vi "Stop All Channels streaming.vi"(1 "Template Refs":refnum<vi>[](array[refnum]), 2 "Handle":i32, 3 "LMMeasurementLib.ICoLMMeasurement":refnum<k7>) -> (0 "error out":errorcluster)   [LabVIEW 2017, in "Powermeter_library.lvlib"]
uses:
  Powermeter_library.lvlib
  Channel States.ctl
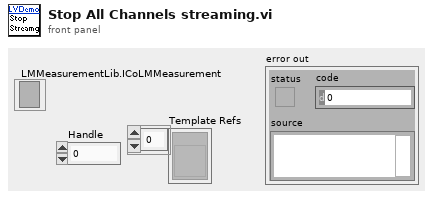
[diagram p1: front panel]
types:
  T1 = typedef "Powermeter_library.lvlib/Channel States.ctl" = enum16{"Init", "Poll", "Set Handle", "Measure"}
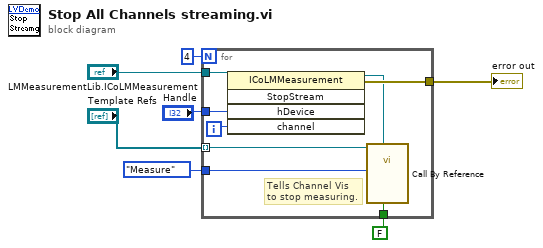
[diagram p0: block diagram]
diagram:
  n1 = for {
    N: 4 -> [_]
    tunnel: "LMMeasurementLib.ICoLMMeasurement" -> [w15]
    tunnel: "Handle" -> [w14]
    tunnel: [w13] -> w3
    tunnel: FALSE -> [w11]
    tunnel: Channel_States."Measure" ("State") -> [w9]
    tunnel: "Template Refs" -> [w8] mode=indexing
    i -> [w12]
    # "Tells Channel Vis to stop measuring."
    n2 = invoke class="ICoLMMeasurement" method="StopStream"(reference=w15, "hDevice"=w14, "channel"=w12) -> (reference out=w10:refnum<k7>, error out=w13:errorcluster)  [unwired: 2 in, 3 out]
    n3 = call-by-ref "?"(reference=w8, "Set Meas"=w11, "OphirLMMeasurementLib.ICoLMMeasurement"=w10, "State"=w9) -> ()  [unwired: 8 in, 3 out]
  }
  "error out" <- w3
